vi "SS Class Init.vi"(7 "VI Refnum":refnum<vi>, 8 "error in (no error)":errorcluster, 9 "Init Data":variant, 10 "Device":string, 11 "Subsystem Filter Wheel in":refnum<class "Subsystem Filter Wheel.lvclass">) -> (0 "error out":errorcluster, 2 "Channel List":refnum<class "HK Item.lvclass">[](array[class]), 3 "Subsystem Filter Wheel out":refnum<class "Subsystem Filter Wheel.lvclass">)   [LabVIEW 2024, in "Subsystem Filter Wheel.lvclass"]
uses:
  Subsystem Filter Wheel.lvclass
  hk-channel-class/hk-channel-class/HK Item/HK Item.lvclass
  Subsystem Class.lvclass
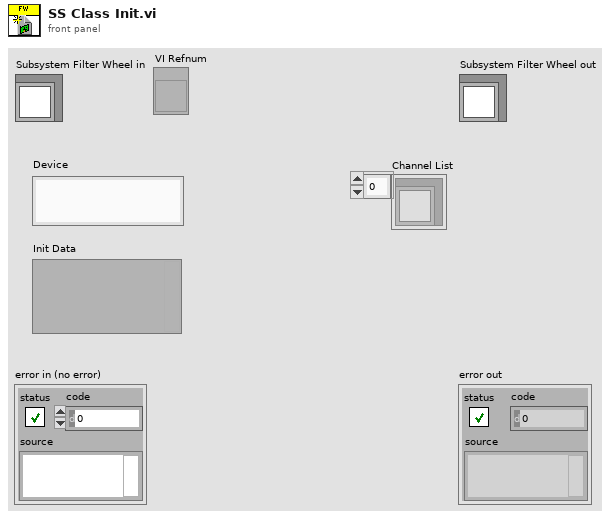
[diagram p1: front panel]
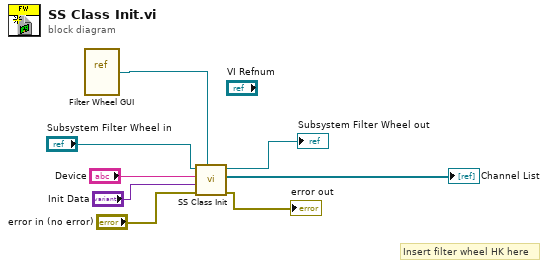
[diagram p0: block diagram]
diagram:
  # "Insert filter wheel HK here"
  n1 = vi-ref "Filter Wheel GUI.vi"() -> (w3:refnum<vi>)
  n2 = call-parent "SS Class Init.vi"("VI Refnum"=w3, "error in (no error)"="error in (no error)", "Init Data"="Init Data", "Device"="Device", "Subsystem Class in"="Subsystem Filter Wheel in") -> ("error out"=→"error out":errorcluster, "Channel List"=→"Channel List":refnum<class "HK Item.lvclass">[], "Subsystem Class out"=→"Subsystem Filter Wheel out":refnum<class "Subsystem Filter Wheel.lvclass">)  [unwired: 4 in]
